vi "Trigger Channel Settings.vi"(6 "Trigger Count (1)":i32=1, 7 "Trigger Point (T: On)":bool=TRUE, 8 "Error In (no error)":errorcluster, 9 "Trigger Mode (1: Continuous)":u16(ring)=1 items=["Hold", "Continuous", "Count"], 10 "Channel (1)":i32=1, 11 "VISA session":refnum<visa-resource-name>) -> (0 "Error Out":errorcluster, 3 "dup VISA session":refnum<visa-resource-name>)   [LabVIEW 2018, in "Agilent PNA Series.lvlib"]
doc: "This VI sets the trigger settings."
uses:
  Agilent PNA Series.lvlib
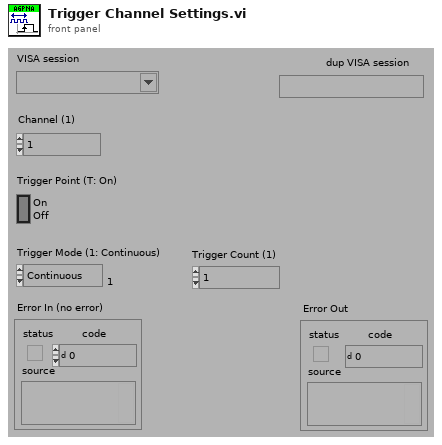
[diagram p1: front panel]
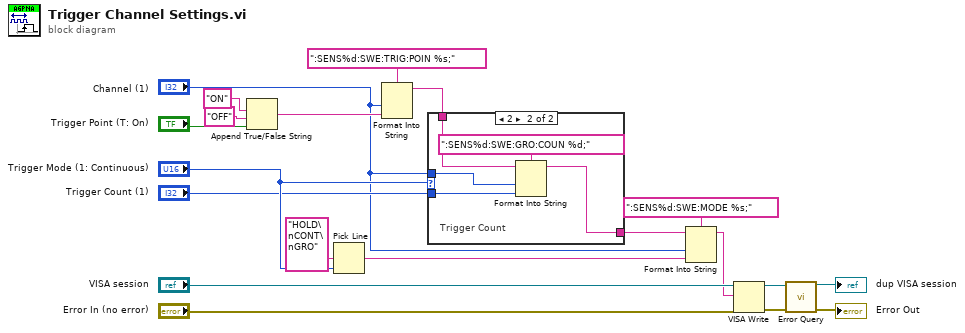
[diagram p0: block diagram]
diagram:
  n1 = Append True/False String(1:"Trigger Point (T: On)", 2:"OFF" ("false string"), 3:"ON" ("true string")) -> (0:w13:string)  [unwired: 1 in]
  n2 = Pick Line(multi-line string="HOLD\nCONT\nGRO", line index="Trigger Mode (1: Continuous)") -> (output string=w6:string)  [unwired: 1 in]
  n3 = Format Into String(format string=":SENS%d:SWE:TRIG:POIN %s;", "Channel (1)", w13) -> (resulting string=w14:string)  [unwired: 2 in, 1 out]
  n4 = case shown="2" "Trigger Mode (1: Continuous)" {
    tunnel: "Channel (1)" -> [_ w25]
    tunnel: "Trigger Count (1)" -> [_ w24]
    tunnel: w14 -> [w21 w23]
    tunnel: [w21 w22] -> w8
    frame 0, Default {
    }
    frame 2 {
      # "Trigger Count"
      n5 = Format Into String(format string=":SENS%d:SWE:GRO:COUN %d;", initial string=w23, w25, w24) -> (resulting string=w22:string)  [unwired: 1 in, 1 out]
    }
  }
  n6 = Format Into String(format string=":SENS%d:SWE:MODE %s;", initial string=w8, "Channel (1)", w6) -> (resulting string=w7:string)  [unwired: 1 in, 1 out]
  n7 = VISA Write(VISA resource name="VISA session", write buffer=w7, error in (no error)="Error In (no error)") -> (VISA resource name out=w4:refnum<visa-resource-name>, error out=w3:errorcluster)  [unwired: 1 out]
  n8 = call "Error Query.vi"("VISA Resource Name"=w4, "error in (no error)"=w3) -> ("VISA Resource Name Out"=→"dup VISA session":refnum<visa-resource-name>, "error out"=→"Error Out":errorcluster)  [unwired: 10 in, 2 out]
